vi "TEST - Get Msg Queue Status.vi"(8 "error in (no error)":errorcluster) -> (0 "error out":errorcluster, 2 "pass":bool)   [LabVIEW 2009]
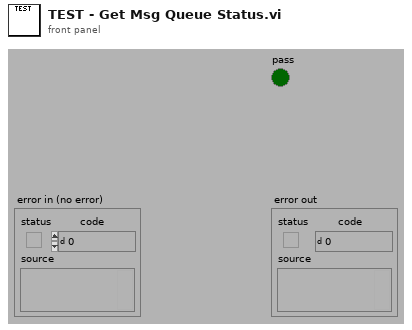
[diagram p1: front panel]
types:
  T1 = typedef "Msg Queue RefNum.ctl" = refnum<k1>
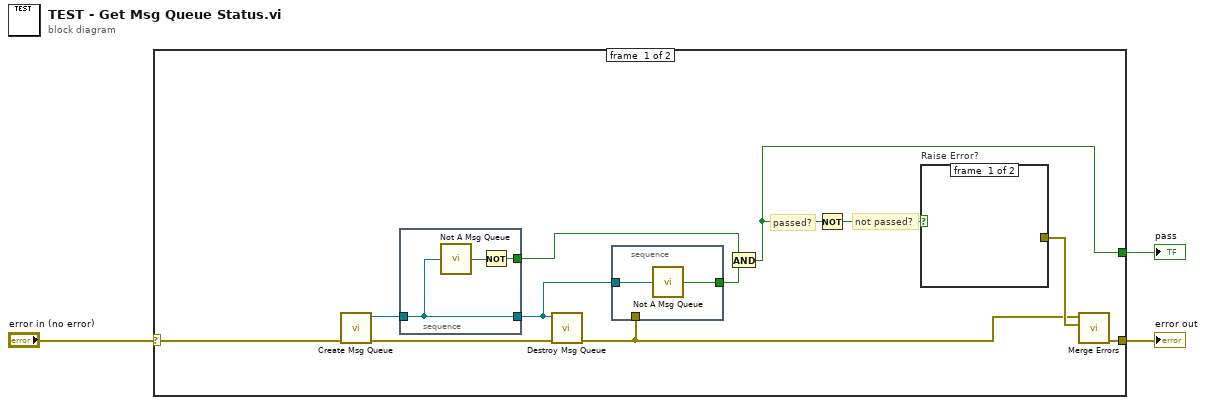
[diagram p0: block diagram]
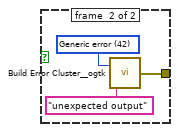
[diagram p2: hidden frame]
diagram:
  n1 = case shown="No Error" "error in (no error)" {
    selector: "error in (no error)" -> [w11 w23]
    tunnel: [w4 _] -> w3
    tunnel: [w14 w23] -> w1
    frame #0 {
      # "not passed?"
      # "passed?"
      n2 = call "Create Msg Queue.vi"("error in (no error)"=w11) -> ("error out"=w9:errorcluster, "msg queue"=w10:T1)  [unwired: 4 in, 1 out]
      n3 = stacked-sequence {
        tunnel: w10 -> [w19]
        tunnel: [w19] -> w8
        tunnel: [w17] -> w6
        frame #0 {
          n4 = call "Not A Msg Queue.vi"("msg queue"=w19) -> ("not a msg queue"=w18:bool)
          n5 = Not(x=w18) -> (.not. x?=w17:bool)
        }
      }
      n6 = call "Destroy Msg Queue.vi"("error in (no error)"=w9, "msg queue"=w8) -> ("error out"=w7:errorcluster)  [unwired: 3 in, 2 out]
      n7 = stacked-sequence {
        tunnel: w8 -> [w16]
        tunnel: w7 -> [_]
        tunnel: [w15] -> w5
        frame #0 {
          n8 = call "Not A Msg Queue.vi"("msg queue"=w16) -> ("not a msg queue"=w15:bool)
        }
      }
      n9 = And(x=w6, y=w5) -> (x .and. y?=w4:bool)
      n10 = Not(x=w4) -> (.not. x?=w12:bool)
      n11 = case "Raise Error?" shown="True" w12 {
        tunnel: [_ w20] -> w13
        frame #0 {
        }
        frame #1 {
          w21 = 42 items=["No error", "Argument error", "Memory is full", "Out of zone", "End of file", "File already open", "Generic file I/O error", "File not found", "File permission error", "Disk is full", "Duplicate path", "Too many files open", "System feature not enabled", "Resource file not found", "Cannot add resource", "Resource not found", "Image not found", "Image memory error", "Pen does not exist", "Config type invalid", "Config token not found", "Config parse error", "Config memory error", "Bad external code format", "Bad external code offset", "External code not present", "Null window", "Destroy window error", "Null menu", "Print aborted", "Bad print record", "Print driver error", "Windows error during printing", "Memory error during printing", "Print dialog error", "Generic print error", "Invalid device refnum", "Device not found", "Device parameter error", "Device unit error", "Cannot open device", "Device call aborted", "Generic error", "Cancelled by user", "Object ID too low", "Object ID too high", "Object not in heap", "Unknown heap", "Unknown object (invalid DefProc)", "Unknown object (DefProc not in table)", "Message out of range", "Invalid (null) method", "Unknown message", "Manager call not supported", "Bad address", "Network operation in progress", "Network operation timed out", "Connection is busy", "Network attribute not supported", "Network error", "Address in use", "System out of memory", "Connection aborted", "Connection refused", "Not connected", "Already connected", "Connection closed", "Initialization error (interapplication manager)", "Bad occurrence", "Wait on unbound occurrence handler", "Occurrence queue overflow", "Datalog type conflict", "Unused", "Unrecognized type (interapplication manager)", "Memory corrupt", "Failed to make temporary DLL", "Old CIN version", "Drag socket not found", "Failed to load drop-object", "Failed to register OLE object", "Failed to release OLE object", "Format specifier type mismatch", "Unknown format specifier", "Too few format specifiers", "Too many format specifiers", "Scan failed", "Newer CIN version", "Error converting to variant", "Runtime menu error", "Password tampered", "Variant attribute not found", "Incompatible variant data type", "Event data is not available", "Event Store is not present", "Occurrence is not found", "Event Queue is not created", "Event info is not available", "Refnum passed is NULL", "Error retrieving Class GUID", "Error retrieving CoClass GUID", "Error retrieving TypeLib GUID.", "Bad built application magic bytes.", "Specific driver is different from the specific driver associated with the Logical Name.", "There is no session opened to the class driver.", "Max Error", "MAX - Error with config objects", "MAX - Error loading configuration", "MAX - Group not supported"]
          n12 = call <userlib>:"Build Error Cluster__ogtk.vi"("String to Prepend to source (\"\")"="unexpected output" ("String to Prepend to source (\"\")"), "code"=w21) -> ("error out"=w20:errorcluster)
        }
      }
      n13 = call <vilib>:"Merge Errors.vi"("error in 2 (no error)"=w13, "error in 1 (no error)"=w7) -> ("error out"=w14:errorcluster)  [unwired: 5 in]
    }
    frame #1 {
    }
  }
  "pass" <- w3
  "error out" <- w1
